vi "CRYunit convert.vi"(11 "A data for units":T1={"Name"="", "Curve"=[], "X data"=1, "Y data"=1, "Z data"=1, "X axis"=0, "Y axis"=1, "Z axis"=1, "X unit"="Hz", "Y unit"="", "Z unit"="deg.", "X dB ref"=1.0, "Y dB ref"=1.0, "Z dB ref"=1.0, "single val"=FALSE, "protected"=FALSE, "display X"=TRUE, "display Y"=TRUE, "display Z"=TRUE, "Test Info"="", "Step No."=0, "Plot Settings"={"Color"=0, "Interpolation"=0, "Point Style"=0, "Line Style"=0, "Point Color"=0, "Line Width"=0, "Bar Plot Style"=0, "Fill To"=0}, "AutoProtect"=FALSE} {"Z data" items=["dB", "Lin"]; "X data" items=["dB", "Lin"]; "Y data" items=["dB", "Lin"]; "Z dB ref" format="%.1f"; "Z axis" items=["Log", "Lin"]; "X dB ref" format="%.1f"; "X axis" items=["Log", "Lin"]; "Y axis" items=["Log", "Lin"]; "Y dB ref" format="%.1f"; "Curve"."z" format="%.2f"; "Curve"."y" format="%.2f"; "Curve"."x" format="%.2f"}) -> (3 "Result out":T1={"Name"="", "Curve"=[], "X data"=1, "Y data"=1, "Z data"=1, "X axis"=0, "Y axis"=1, "Z axis"=1, "X unit"="Hz", "Y unit"="", "Z unit"="deg.", "X dB ref"=1.0, "Y dB ref"=1.0, "Z dB ref"=1.0, "single val"=FALSE, "protected"=FALSE, "display X"=TRUE, "display Y"=TRUE, "display Z"=TRUE, "Test Info"="", "Step No."=0, "Plot Settings"={"Color"=0, "Interpolation"=0, "Point Style"=0, "Line Style"=0, "Point Color"=0, "Line Width"=0, "Bar Plot Style"=0, "Fill To"=0}, "AutoProtect"=FALSE} {"Z data" items=["dB", "Lin"]; "X data" items=["dB", "Lin"]; "Y data" items=["dB", "Lin"]; "Z dB ref" format="%.1f"; "Z axis" items=["Log", "Lin"]; "X dB ref" format="%.1f"; "X axis" items=["Log", "Lin"]; "Y axis" items=["Log", "Lin"]; "Y dB ref" format="%.1f"; "Curve"."z" format="%.2f"; "Curve"."y" format="%.2f"; "Curve"."x" format="%.2f"})   [LabVIEW 2013]
uses:
  Typedef Control/CRYData Cluster.ctl
  CRYPost Processing Global.vi
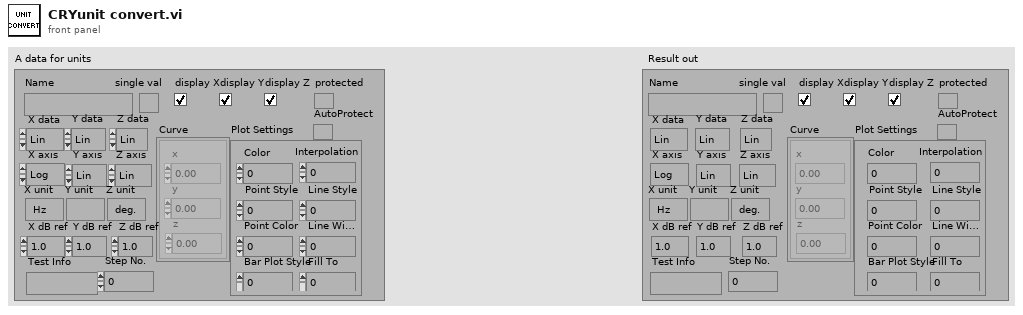
[diagram p1: front panel]
types:
  T1 = typedef "CRYData Cluster.ctl" = cluster{"Name":string, "Curve":cluster{"x":dbl, "y":dbl, "z":dbl}[], "X data":u16, "Y data":u16, "Z data":u16, "X axis":u16, "Y axis":u16, "Z axis":u16, "X unit":string, "Y unit":string, "Z unit":string, "X dB ref":dbl, "Y dB ref":dbl, "Z dB ref":dbl, "single val":bool, "protected":bool, "display X":bool, "display Y":bool, "display Z":bool, "Test Info":string, "Step No.":i32, "Plot Settings":cluster{"Color":u32, "Interpolation":u8, "Point Style":u8, "Line Style":u8, "Point Color":u32, "Line Width":u8, "Bar Plot Style":u8, "Fill To":i16}, "AutoProtect":bool}
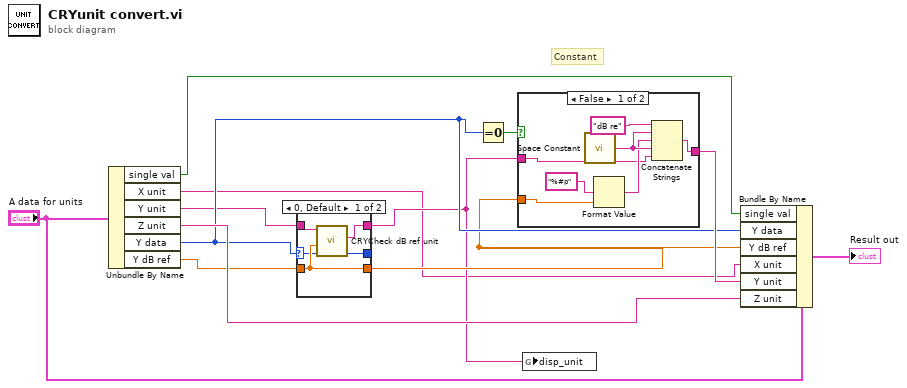
[diagram p0: block diagram]
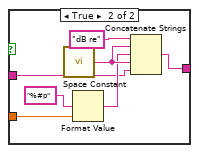
[diagram p3: hidden frame]
diagram:
  # "Constant"
  n1 = Unbundle By Name("A data for units") -> ("single val"=w2:bool, "X unit"=w1:string, "Y unit"=w4:string, "Z unit"=w12:string, "Y data"=w6:u16, "Y dB ref"=w7:dbl)
  n2 = case shown="0, Default" w6 {
    selector: w6 -> [w13 w17]
    tunnel: w4 -> [w16 w19]
    tunnel: [w15 w19] -> w3
    tunnel: w7 -> [w14 w18]
    tunnel: [w14 w18] -> w5
    tunnel: [w13 w17] -> _
    frame 0, Default {
      n3 = call "CRYCheck dB ref unit.vi"("dB ref in"=w14, "Unit in"=w16) -> ("Lin unit out"=w15:string)  [unwired: 9 out]
    }
    frame 1 {
    }
  }
  n4 = Equal To 0?(x=w6) -> (x = 0?=w9:bool)
  n5 = case shown="False" w9 {
    tunnel: w3 -> [w22 w28]
    tunnel: [w20 w27] -> w8
    tunnel: w5 -> [w21 w32]
    frame False {
      n6 = call <vilib>:"Space Constant.vi"() -> ("String"=w25:string)
      n7 = Format Value(format string="%#p", value (0)=w21) -> (output string=w23:string)  [unwired: 1 out]
      n8 = Concatenate Strings("dB re" ("string"), w25, w23, w25, w22) -> (w20:string)
    }
    frame True {
      n9 = call <vilib>:"Space Constant.vi"() -> ("String"=w31:string)
      n10 = Format Value(format string="%#p", value (0)=w32) -> (output string=w29:string)  [unwired: 1 out]
      n11 = Concatenate Strings("dB re" ("string"), w31, w29, w31, w28) -> (w27:string)
    }
  }
  n12 = global write "CRYPost Processing Global.vi" "disp_unit"(w3) -> ()
  n13 = Bundle By Name(cluster="A data for units", "single val"=w2, "Y data"=w6, "Y dB ref"=w5, "X unit"=w1, "Y unit"=w8, "Z unit"=w12) -> (→"Result out":T1)
